vi "Process ILC Data.vi"(8 "error in (no error)":errorcluster, 11 "Model in":refnum<class "Model.lvclass">) -> (0 "error out":errorcluster, 3 "Model out":refnum<class "Model.lvclass">)   [LabVIEW 2015, in "Model.lvclass"]
uses:
  Model.lvclass
  Model.lvclass/Model.ctl
  Common_RT_FAILC/FAILC/FAILC.lvclass/FAILC.ctl
  Common_RT_FAILC/FAILC/FAILC.lvclass
  Calculators/Cylinder To Actuator Forces/Cylinder To Actuator Forces.lvclass
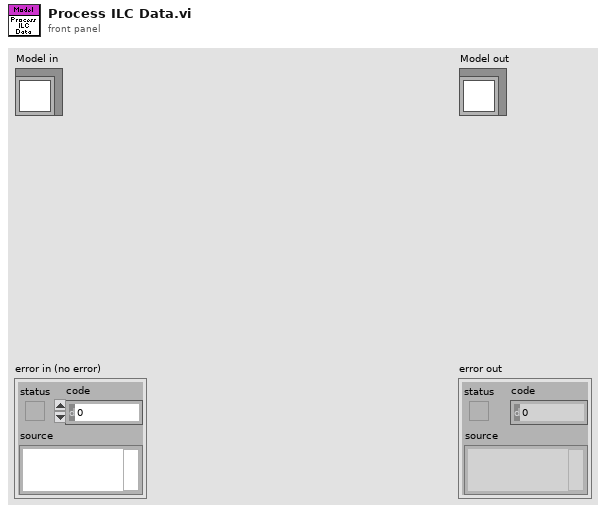
[diagram p1: front panel]
types:
  T1 = typedef "RTFAILC.lvlib/FAData.ctl" = cluster{"FAConstants":T2, "FACommand":T3, "FATelemetry":T5, "FAResponses":T6}
  T2 = typedef "RTFAILC.lvlib/FAConstants.ctl" = cluster{"ID":i16}
  T3 = typedef "RTFAILC.lvlib/FACommand.ctl" = cluster{"AxialSetPoint":i32, "LateralSetPoint":i32, "PressureServoValveSettings":T4, "BoosterValveSettings":T4}
  T4 = typedef "RTFAILC.lvlib/FAPID.ctl" = cluster{"Kp":sgl, "Ki":sgl, "Kd":sgl, "Kf":sgl}
  T5 = typedef "RTFAILC.lvlib/FATelemetry.ctl" = cluster{"ILCFault":bool, "BroadcastCounter":u8, "AxialLoadCellForce":sgl, "LateralLoadCellForce":sgl, "AxialPressure":T4, "AxialTurbo":T4, "LateralPressure":T4, "LateralTurbo":T4}
  T6 = typedef "RTFAILC.lvlib/FAResponses.ctl" = cluster{"PIDParameters":T7, "ReadPIDParameters":T7, "SetForce":T7, "ForceAndStatus":T7}
  T7 = typedef "RTModbus.lvlib/ExceptionCodes.ctl" = u16
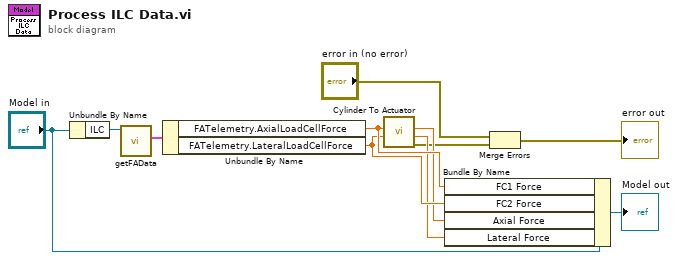
[diagram p0: block diagram]
diagram:
  n1 = Unbundle By Name("Model in") -> ("ILC"=w10:refnum<class "FAILC.lvclass">)
  n2 = call "getFAData.vi"("FAILC in"=w10) -> ("FAData"=w11:T1)  [unwired: 9 in, 1 out]
  n3 = Unbundle By Name(w11) -> ("FATelemetry.AxialLoadCellForce"=w8:sgl, "FATelemetry.LateralLoadCellForce"=w7:sgl)
  n4 = call "Cylinder To Actuator.vi"("FC2 Measured Value"=w7, "FC1 Measured Value"=w8) -> ("error out"=w4:errorcluster, "Lateral Force"=w5:dbl, "Axial Force"=w6:dbl)  [unwired: 6 in, 1 out]
  n5 = Bundle By Name(cluster="Model in", "FC1 Force"=w8, "FC2 Force"=w7, "Axial Force"=w6, "Lateral Force"=w5) -> (→"Model out":refnum<class "Model.lvclass">)
  n6 = Merge Errors("error in (no error)", w4) -> (→"error out":errorcluster)
